vi "Accessor Discription.vi"(8 "error in (no error)":errorcluster, 10 "Read/Write(T->Read)":bool, 11 "VI":refnum<vi>) -> (0 "error out":errorcluster, 2 "VI Description":string, 3 "VI out":refnum<vi>)   [LabVIEW 2014]
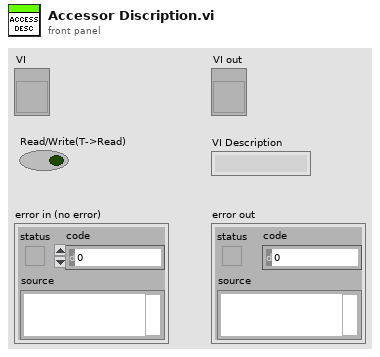
[diagram p1: front panel]
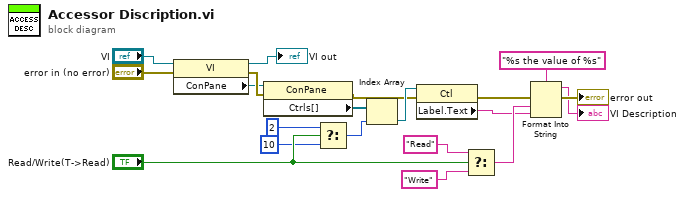
[diagram p0: block diagram]
diagram:
  n1 = property class="VI"(reference="VI", error in="error in (no error)") -> (reference out=→"VI out":refnum<vi>, error out=w14:errorcluster, "ConPane"=w11:refnum<vi>)
  n2 = property class="ConPane"(reference=w11, error in=w14) -> (error out=w4:errorcluster, "Ctrls[]"=w10:refnum<vi>[])  [unwired: 1 out]
  n3 = Select(t=2 ("index"), s="Read/Write(T->Read)", f=10) -> (s? t:f=w6:i32)
  n4 = Index Array(array=w10, index=w6) -> (element=w5:refnum<vi>)
  n5 = property class="Ctl"(reference=w5, error in=w4) -> (error out=w1:errorcluster, "Label.Text"=w3:string)  [unwired: 1 out]
  n6 = Select(t="Read" ("VI Description"), s="Read/Write(T->Read)", f="Write" ("VI Description")) -> (s? t:f=w18:string)
  n7 = Format Into String(format string="%s the value of %s", error in=w1, w18, w3) -> (resulting string=→"VI Description":string, error out=→"error out":errorcluster)  [unwired: 1 in]
